vi "Apply.vi"(8 "error in (no error)":errorcluster, 11 "Scope PXI Base CFG in":refnum<class "Scope PXI Base CFG.lvclass">) -> (0 "error out":errorcluster, 3 "Scope PXI Base CFG out":refnum<class "Scope PXI Base CFG.lvclass">)   [LabVIEW 2023, in "Scope PXI Base CFG.lvclass"]
uses:
  Scope PXI Base CFG.lvclass
  Scope PXI Base CFG.lvclass/Scope PXI Base CFG.ctl
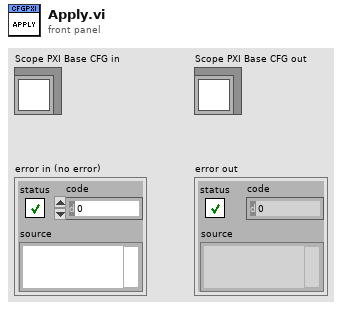
[diagram p1: front panel]
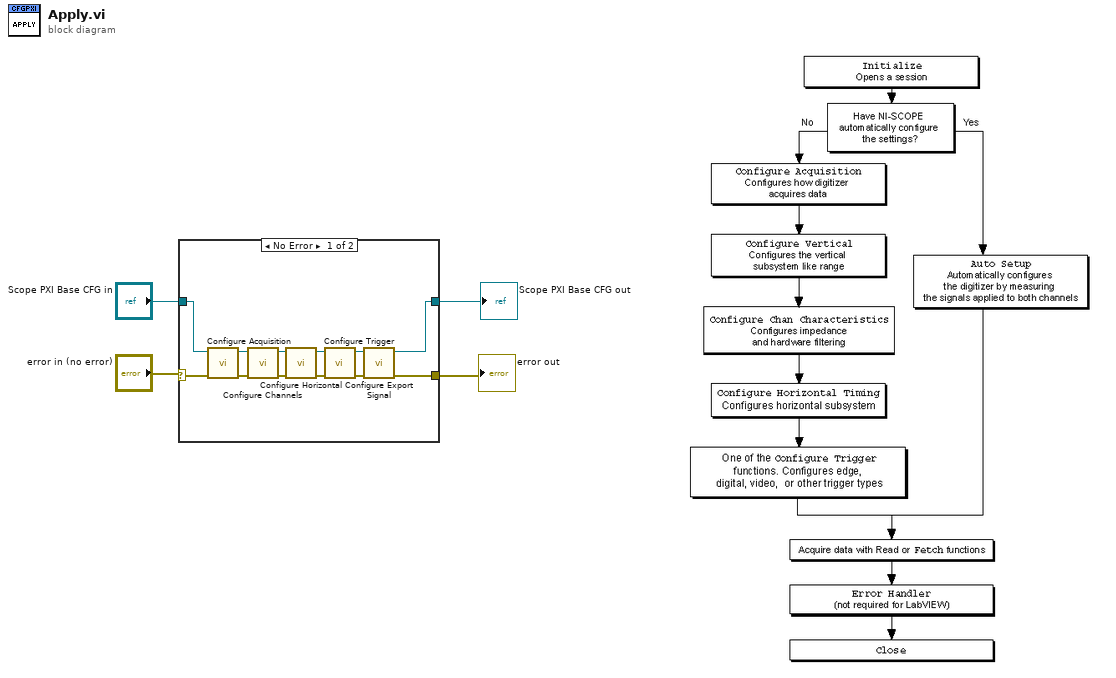
[diagram p0: block diagram]
diagram:
  n1 = case shown="No Error" "error in (no error)" {
    selector: "error in (no error)" -> [w16 w18]
    tunnel: "Scope PXI Base CFG in" -> [w15 w17]
    tunnel: [w6 w17] -> w2
    tunnel: [w5 w18] -> w1
    frame No Error {
      n2 = call-dynamic "Configure Acquisition.vi"("error in (no error)"=w16, "Scope PXI Base CFG in"=w15) -> ("error out"=w14:errorcluster, "Scope PXI Base CFG out"=w13:refnum<class "Scope PXI Base CFG.lvclass">)  [unwired: 8 in]
      n3 = call-dynamic "Configure Channels.vi"("error in"=w14, "Scope PXI Base CFG in"=w13) -> ("error out"=w12:errorcluster, "Scope PXI Base CFG out"=w11:refnum<class "Scope PXI Base CFG.lvclass">)  [unwired: 8 in]
      n4 = call-dynamic "Configure Horizontal.vi"("error in"=w12, "Scope PXI Base CFG in"=w11) -> ("error out"=w10:errorcluster, "Scope PXI Base CFG out"=w9:refnum<class "Scope PXI Base CFG.lvclass">)  [unwired: 8 in]
      n5 = call-dynamic "Configure Trigger.vi"("error in"=w10, "Scope PXI Base CFG in"=w9) -> ("error out"=w8:errorcluster, "Scope PXI Base CFG out"=w7:refnum<class "Scope PXI Base CFG.lvclass">)  [unwired: 8 in]
      n6 = call-dynamic "Configure Export Signal.vi"("error in"=w8, "Scope PXI Base CFG in"=w7) -> ("error out"=w5:errorcluster, "Base CFG out"=w6:refnum<class "Scope PXI Base CFG.lvclass">)  [unwired: 8 in]
    }
    frame Error {
    }
  }
  "error out" <- w1
  "Scope PXI Base CFG out" <- w2
